vi "DB_MAIN.vi"(11 "Message Queues":T1) -> ()   [LabVIEW 2024]
uses:
  ARCH/Message Queue/All Message Queues.ctl
  ARCH/Message Queue/Message Cluster.ctl
  CAM/SRC/CTRLS/CAM module Data.ctl
  CTRLS/Main Tabs.ctl
  CTRLS/Serials DB Operations Enum.ctl
  CTRLS/Serial status Enum.ctl
  CTRLS/run statistics.ctl
  CTRLS/Workorder DB operation enum.ctl
  CTRLS/Workorder status enum.ctl
  CTRLS/Open Batch Data.ctl
  CTRLS/GLB_VAR.vi
  ARCH/Message Queue/Message Queue.lvlib
  Printer/Domino LM.lvlib
  CAM/RSeries_CAM.lvlib
panel:
  out "error out":errorcluster
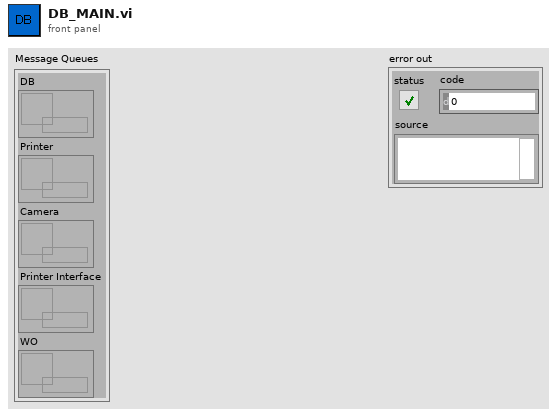
[diagram p1: front panel]
types:
  T1 = typedef "All Message Queues.ctl" = cluster{"DB":refnum<queue>, "Printer":refnum<queue>, "Camera":refnum<queue>, "Printer Interface":refnum<queue>, "WO":refnum<queue>}
  T2 = typedef "Message Queue.lvlib/Message Cluster.ctl" = cluster{"Message":string, "Message Data":variant}
  T3 = typedef "CAM module Data.ctl" = cluster{"IP":string, "sending Port ":u32, "BatchData":refnum<vi>, "Recieveing Port":u32, "Caller Quue":refnum<queue>}
  T4 = cluster{"Subscriber Message":string, "Subscribe Queue":refnum<queue>}
  T5 = typedef "Main Tabs.ctl" = enum32{"Login", "Main", "woManagement", "Settings", "Home"}
  T6 = enum8{"Enabled", "Disabled", "Disabled and Grayed Out"}
  T7 = enum16{"Init SRL Buffer", "Insert SRL in Buffer", "Insert SRL Status", "Remove SRL from Buffer", "pop serial"}
  T8 = typedef "Serial status Enum.ctl" = enum16{"NOT USED", "PRINTED", "ACCEPTED", "REJECTED"}
  T9 = typedef "Serials DB Operations Enum.ctl" = enum16{"Update serial verify status", "Get serials Based on Status", "Insert serials", "Update serial print status", "Get all Batch Serials", "Get Serial Status"}
  T10 = enum16{"Init SRL Buffer", "Insert SRL in Buffer", "Insert SRL Status", "Remove SRL from Buffer"}
  T11 = typedef "run statistics.ctl" = cluster{"Good":dbl, "Bad":dbl, "Good %":dbl, "Bad %":dbl}
  T12 = typedef "Workorder DB operation enum.ctl" = enum16{"Get Open Workorder", "Change WO Status", "Create WO", "Get ready and paused WOs"}
  T13 = typedef "Workorder status enum.ctl" = enum16{"Open", "Ready", "On Hold", "Closed"}
  T14 = typedef "Open Batch Data.ctl" = cluster{"Batch Name":string, "Batch Number":string, "GTIN":string, "Expiry Date":string, "MFG Date":string}
  T15 = typedef "REF.ctl" = cluster{"Save Settings":refnum<vi>, "Navigation":refnum<vi>, "Main Tab":refnum<vi>, "Password":refnum<vi>, "BatchData":refnum<vi>, "Serial Data":refnum<vi>, "Username":refnum<vi>, "Stop Printing":refnum<vi>, "Run statistics":refnum<vi>, "System settings":refnum<vi>, "Batch Managment contol":refnum<vi>, "Start Printing":refnum<vi>, "BatchData MNG":refnum<vi>, "MSG Cenetr":refnum<vi>, "Printer status":refnum<vi>, "Printer Message Config":refnum<vi>, "Ready and Paused Batches":refnum<vi>, "Camera Setup":refnum<vi>, "Batch statistics":refnum<vi>, "Logout":refnum<vi>}
  T16 = typedef "System settings.ctl" = cluster{"Machine IP":string, "Camera IP":string, "Printer IP":string, "Scanner settings":string, "Server Path":path, "Sending Port":u32, "Recieveing Port":u32}
  T17 = cluster{"DM Text":string, "GTIN":string, "Batch":string, "Expiry Date":string, "MFG Date":string, "Serial Number":string, "SSCC":string}
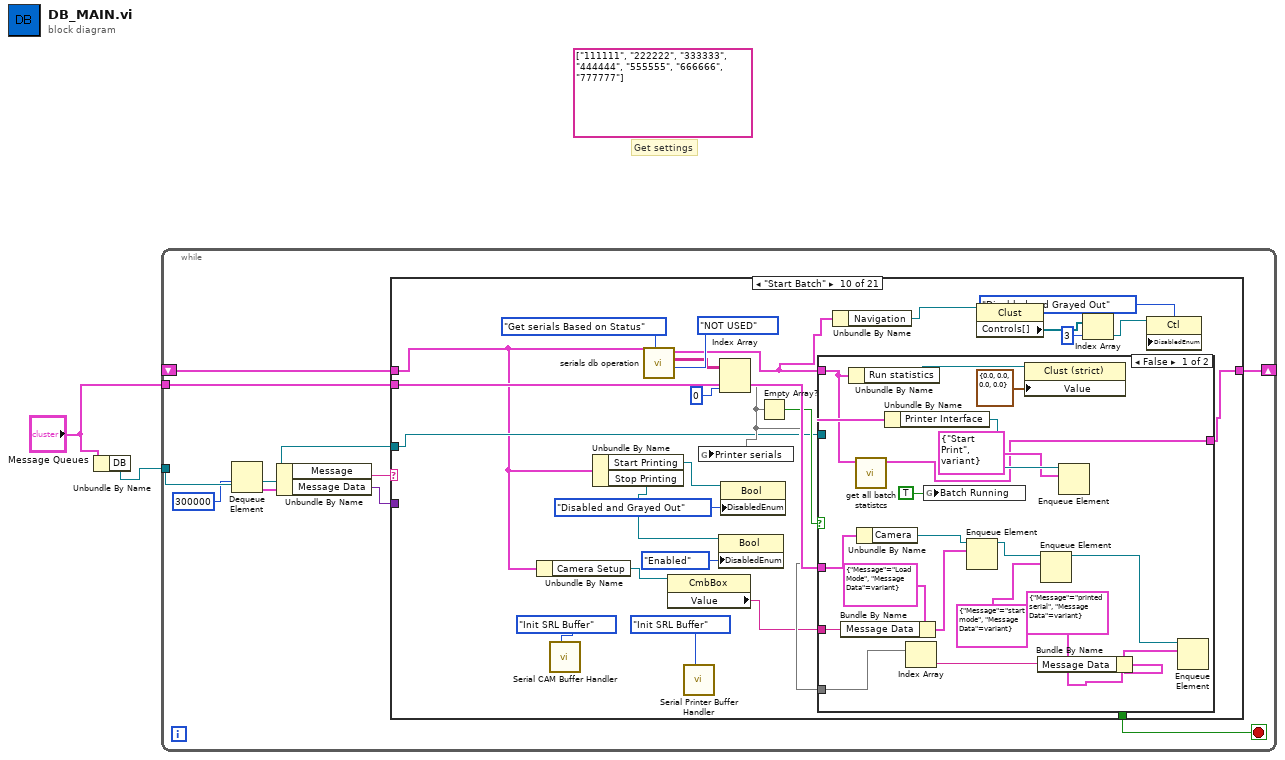
[diagram p0: block diagram]
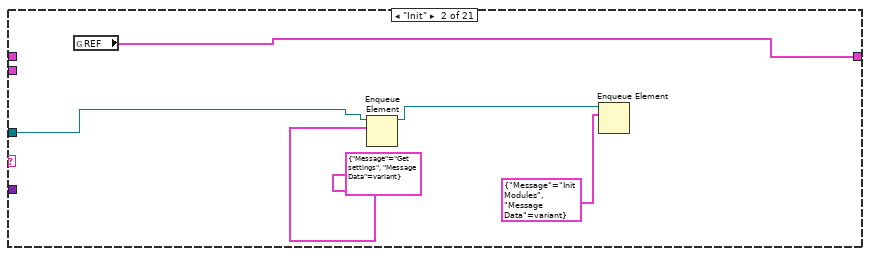
[diagram p3: hidden frame]
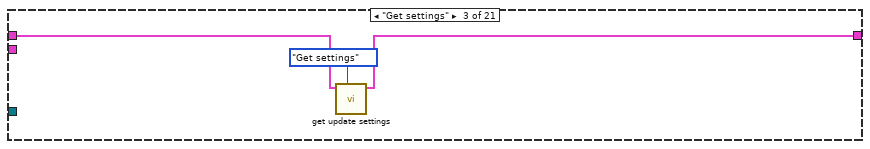
[diagram p4: hidden frame]
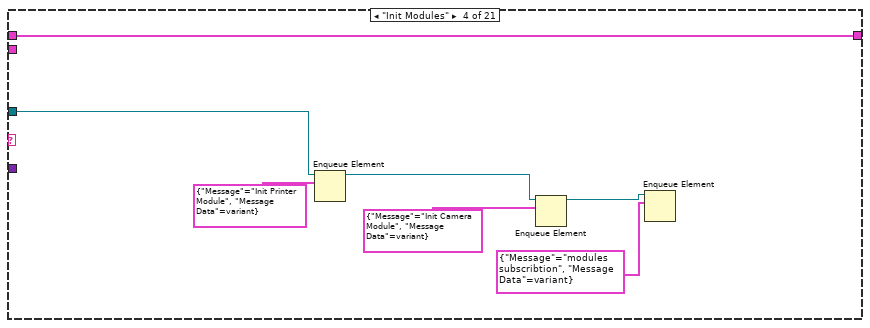
[diagram p5: hidden frame]
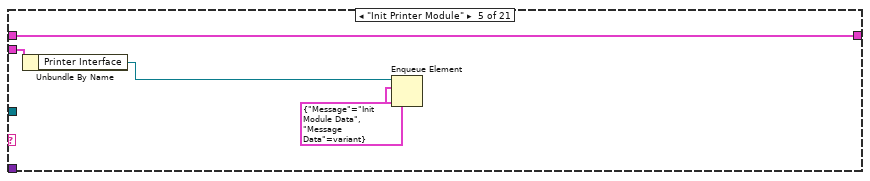
[diagram p6: hidden frame]
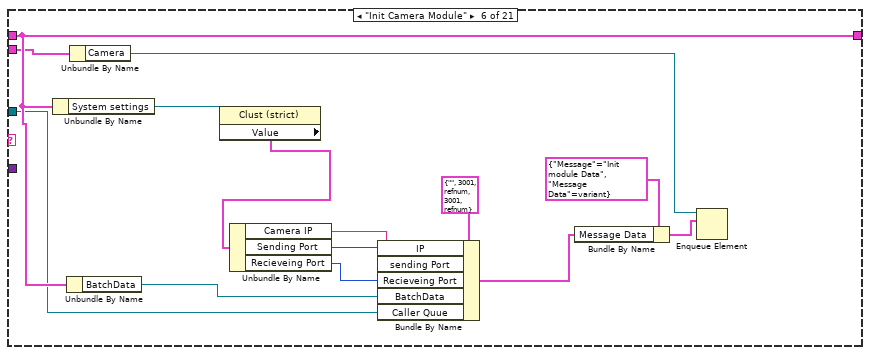
[diagram p7: hidden frame]
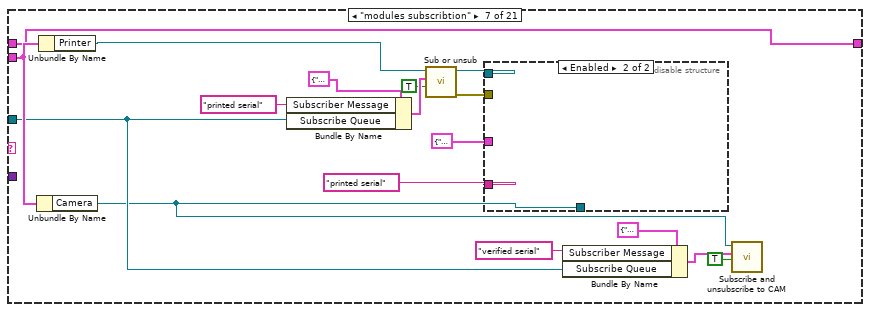
[diagram p8: hidden frame]
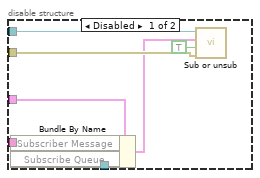
[diagram p9: hidden frame]
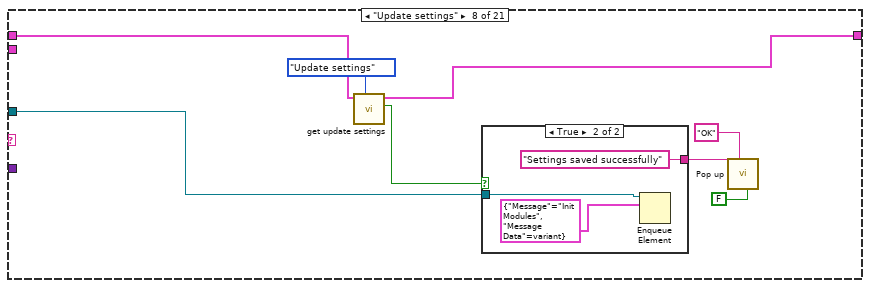
[diagram p10: hidden frame]
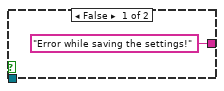
[diagram p11: hidden frame]
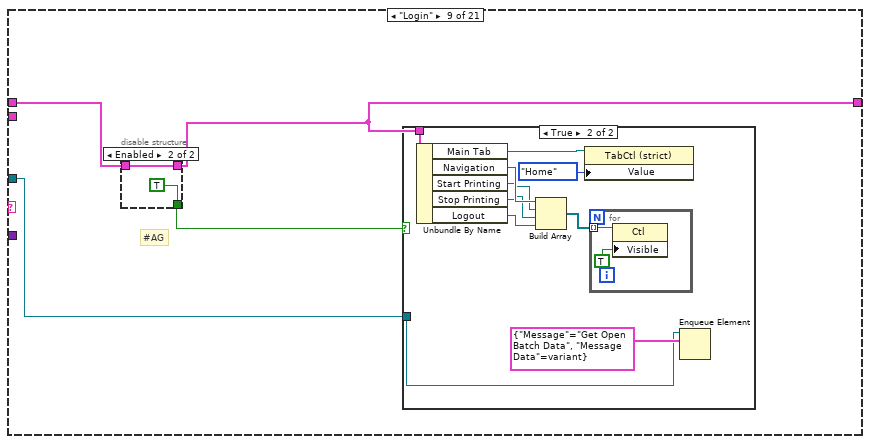
[diagram p12: hidden frame]
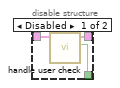
[diagram p13: hidden frame]
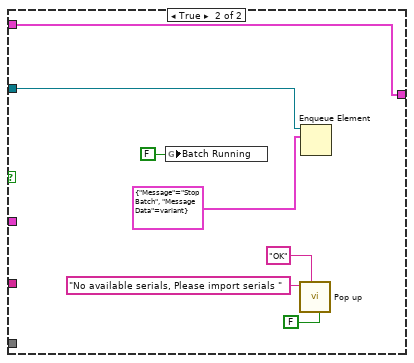
[diagram p15: hidden frame]
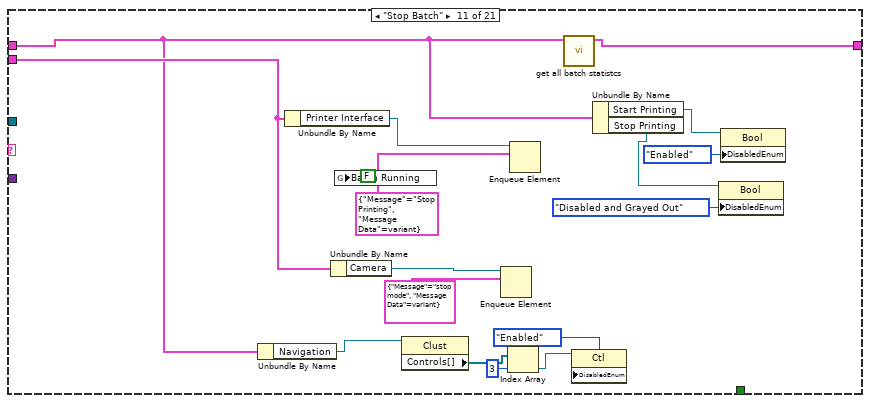
[diagram p16: hidden frame]
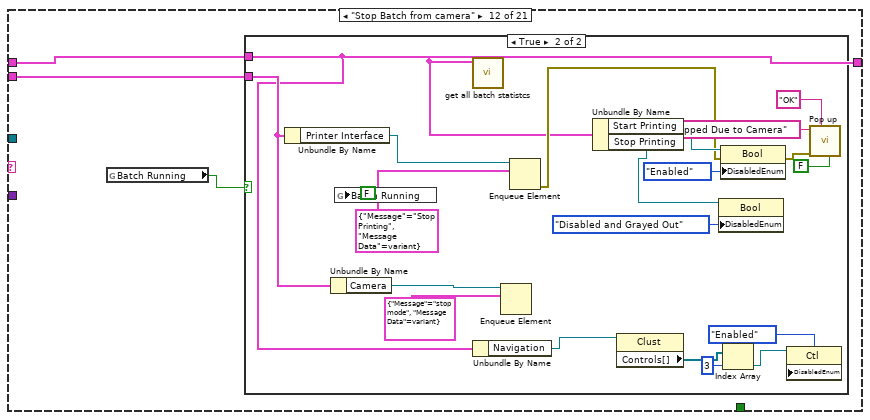
[diagram p17: hidden frame]
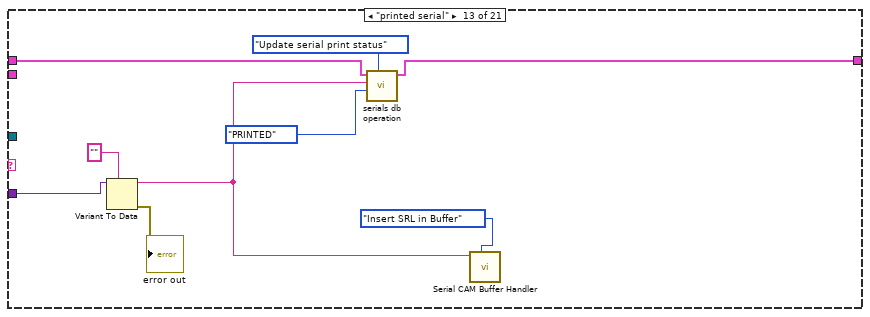
[diagram p19: hidden frame]
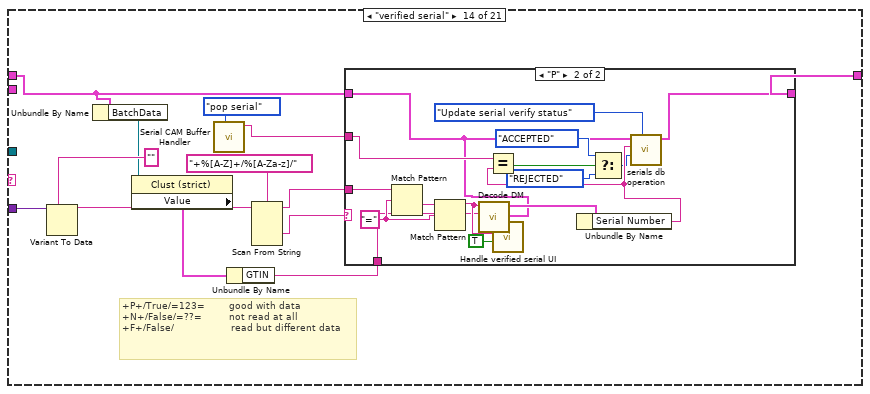
[diagram p20: hidden frame]
diagram:
  (unwired) string[] ["111111", "222222", "333333", "444444", "555555", "666666", "777777"] ("Printer serials")
  # "Get settings"
  n1 = Unbundle By Name("Message Queues") -> ("DB"=w2:refnum<queue>)
  n2 = while {
    tunnel: w2 -> [w12]
    tunnel: "Message Queues" -> [w5]
    shift-right: [w4] -> _
    shift-left: _ -> [w3]
    stop <- w7 stop-if-true
    n3 = Dequeue Element(queue=w12, timeout in ms (-1)=300000) -> (queue out=w8:refnum<queue>, element=w11:T2)  [unwired: 1 in, 2 out]
    n4 = Unbundle By Name(w11) -> ("Message"=w10:string, "Message Data"=w9:variant)
    n5 = case shown="\"Start Batch\"" w10 {
      tunnel: w9 -> [_ _ _ _ _ _ _ _ _ _ _ _ w199 w215 _ _ _ _ _ _ _]
      tunnel: w8 -> [_ w17 _ w28 _ w33 w49 w71 w86 w114 _ _ _ _ _ w275 _ w321 w340 w351 _]
      tunnel: [_ _ _ _ _ _ _ _ _ _ _ _ _ _ _ _ _ _ _ _ TRUE] -> w7
      tunnel: w5 -> [_ _ _ _ w32 w35 w54 _ _ w121 w155 w173 _ _ _ _ _ _ _ _ _]
      tunnel: [w13 w14 w20 w22 w29 w39 w53 w77 w84 w110 w161 w172 w202 w210 w264 w280 w306 w322 w344 w354 w360] -> w4
      tunnel: w3 -> [w13 _ w21 w22 w29 w39 w53 w78 w85 w113 w154 w172 w203 w207 w272 w278 w305 w320 w346 w353 w360]
      frame Default {
      }
      frame "Init" {
        n6 = global read "GLB_VAR.vi" "REF"() -> (w14:T15)
        n7 = Enqueue Element(queue=w17, element=T2 {"Message"="Get settings", "Message Data"=variant}) -> (queue out=w15:refnum<queue>)  [unwired: 2 in, 2 out]
        n8 = Enqueue Element(queue=w15, element=T2 {"Message"="Init Modules", "Message Data"=variant}) -> ()  [unwired: 2 in, 3 out]
      }
      frame "Get settings" {
        n9 = call "get update settings.vi"("settings DB OP"=enum16{"Get settings", "Update settings"}."Get settings", "REF in"=w21) -> ("REF out"=w20:T15)  [unwired: 7 in, 2 out]
      }
      frame "Init Modules" {
        n10 = Enqueue Element(queue=w28, element=T2 {"Message"="Init Printer Module", "Message Data"=variant}) -> (queue out=w25:refnum<queue>)  [unwired: 2 in, 2 out]
        n11 = Enqueue Element(queue=w25, element=T2 {"Message"="Init Camera Module", "Message Data"=variant}) -> (queue out=w24:refnum<queue>)  [unwired: 2 in, 2 out]
        n12 = Enqueue Element(queue=w24, element=T2 {"Message"="modules subscribtion", "Message Data"=variant}) -> ()  [unwired: 2 in, 3 out]
      }
      frame "Init Printer Module" {
        n13 = Unbundle By Name(w32) -> ("Printer Interface"=w31:refnum<queue>)
        n14 = Enqueue Element(queue=w31, element=T2 {"Message"="Init Module Data", "Message Data"=variant}) -> ()  [unwired: 2 in, 3 out]
      }
      frame "Init Camera Module" {
        n15 = Unbundle By Name(w39) -> ("System settings"=w41:refnum<vi>)
        n16 = Unbundle By Name(w39) -> ("BatchData"=w37:refnum<vi>)
        n17 = Unbundle By Name(w35) -> ("Camera"=w34:refnum<queue>)
        n18 = property class="Clust (strict)"(reference=w41) -> ("Value"=w40:T16)  [unwired: 1 in, 2 out]
        n19 = Unbundle By Name(w40) -> ("Camera IP"=w43:string, "Sending Port"=w44:u32, "Recieveing Port"=w36:u32)
        n20 = Bundle By Name(cluster=T3 {"IP"="", "sending Port "=3001, "BatchData"=refnum, "Recieveing Port"=3001, "Caller Quue"=refnum} ("CAM module Data"), "IP"=w43, "sending Port"=w44, "Recieveing Port"=w36, "BatchData"=w37, "Caller Quue"=w33) -> (w42:T3)
        n21 = Bundle By Name(cluster=T2 {"Message"="Init module Data", "Message Data"=variant} ("element"), "Message Data"=w42) -> (w45:T2)
        n22 = Enqueue Element(queue=w34, element=w45) -> ()  [unwired: 2 in, 3 out]
      }
      frame "modules subscribtion" {
        n23 = Unbundle By Name(w54) -> ("Camera"=w48:refnum<queue>)
        n24 = Unbundle By Name(w54) -> ("Printer"=w55:refnum<queue>)
        n25 = Bundle By Name(cluster=T4 {"Subscriber Message"="", "Subscribe Queue"=refnum} ("Subscriber Data"), "Subscriber Message"="printed serial", "Subscribe Queue"=w49) -> (w62:T4)
        n26 = call "Sub or unsub.vi"("Sub T/ Unsub F"=TRUE, "Subscriber Data"=w62, "Printer"=w55) -> ("error out"=w58:errorcluster, "printer queue out"=w57:refnum<queue>)  [unwired: 7 in]
        n27 = disable-structure shown="Enabled" {
          disable-tunnel: "printed serial" ("Subscriber Message") -> [w70 _]
          disable-tunnel: w58 -> [w69 _]
          disable-tunnel: w57 -> [w68 _]
          disable-tunnel: T4 {"Subscriber Message"="", "Subscribe Queue"=refnum} ("Subscriber Data") -> [w66 _]
          disable-tunnel: w48 -> [w65 _]
          frame Disabled {
            n28 = Bundle By Name(cluster=w66, "Subscriber Message"=w70, "Subscribe Queue"=w65) -> (w67:T4)
            n29 = call "Sub or unsub.vi"("error in (no error)"=w69, "Sub T/ Unsub F"=TRUE, "Subscriber Data"=w67, "Printer"=w68) -> ()  [unwired: 6 in, 2 out]
          }
          frame Enabled {
          }
        }
        n30 = Bundle By Name(cluster=T4 {"Subscriber Message"="", "Subscribe Queue"=refnum} ("Subscriber Data"), "Subscriber Message"="verified serial", "Subscribe Queue"=w49) -> (w50:T4)
        n31 = call "Subscribe and unsubscribe to CAM.vi"("Sub T/ Unsub F"=TRUE, "Subscriber Data"=w50, "Camera Queue"=w48) -> ()  [unwired: 7 in, 2 out]
      }
      frame "Update settings" {
        n32 = call "get update settings.vi"("settings DB OP"=enum16{"Get settings", "Update settings"}."Update settings", "REF in"=w78) -> ("success?"=w75:bool, "REF out"=w77:T15)  [unwired: 7 in, 1 out]
        n33 = case shown="True" w75 {
          tunnel: ["Error while saving the settings!" "Settings saved successfully"] -> w72
          tunnel: w71 -> [_ w80]
          frame False {
          }
          frame True {
            n34 = Enqueue Element(queue=w80, element=T2 {"Message"="Init Modules", "Message Data"=variant}) -> ()  [unwired: 2 in, 3 out]
          }
        }
        n35 = call "Pop up.vi"("Close Visible"=FALSE, "OK Boolean Text"="OK", "Title IN"=w72) -> ()  [unwired: 7 in, 2 out]
      }
      frame "Login" {
        # "#AG"
        n36 = disable-structure shown="Enabled" {
          disable-tunnel: w85 -> [w89 w91]
          disable-tunnel: [w88 w91] -> w84
          disable-tunnel: [w87 TRUE ("Result")] -> w83
          frame Disabled {
            n37 = call "handle user check.vi"("REF"=w89) -> ("Result"=w87:bool, "REF out"=w88:T15)  [unwired: 8 in, 1 out]
          }
          frame Enabled {
          }
        }
        n38 = case shown="True" w83 {
          tunnel: w84 -> [_ w100]
          tunnel: w86 -> [_ w97]
          frame False {
          }
          frame True {
            n39 = Unbundle By Name(w100) -> ("Main Tab"=w99:refnum<vi>, "Navigation"=w96:refnum<vi>, "Start Printing"=w95:refnum<vi>, "Stop Printing"=w94:refnum<vi>, "Logout"=w93:refnum<vi>)
            n40 = Build Array(w96, w95, w94, w93) -> (w92:refnum<vi>[])
            n41 = property on="Property Node" class="TabCtl (strict)"(reference=w99, "Value"=Main_Tabs."Home" ("Main Tab")) -> ()  [unwired: 1 in, 2 out]
            n42 = for {
              tunnel: w92 -> [w102] mode=indexing
              n43 = property on="Property Node" class="Ctl"(reference=w102, "Visible"=TRUE) -> ()  [unwired: 1 in, 2 out]
            }
            n44 = Enqueue Element(queue=w97, element=T2 {"Message"="Get Open Batch Data", "Message Data"=variant}) -> ()  [unwired: 2 in, 3 out]
          }
        }
      }
      frame "Start Batch" {
        n45 = Unbundle By Name(w113) -> ("Camera Setup"=w112:refnum<vi>)
        n46 = call "Serial CAM Buffer Handler.vi"("Serials buffer operations"=T7."Init SRL Buffer") -> ()  [unwired: 8 in, 3 out]
        n47 = Unbundle By Name(w113) -> ("Start Printing"=w120:refnum<vi>, "Stop Printing"=w118:refnum<vi>)
        n48 = call "serials db operation.vi"("SRL DB OP"=Serials_DB_Operations_Enum."Get serials Based on Status", "Status"=Serial_status_Enum."NOT USED", "REF"=w113) -> ("Fetched Serials"=w124:string[][], "REF out"=w109:T15)  [unwired: 5 in, 2 out]
        n49 = property class="CmbBox"(reference=w112) -> ("Value"=w111:string)  [unwired: 1 in, 2 out]
        n50 = call "Serial Printer Buffer Handler.vi"("Serials buffer operations"=T10."Init SRL Buffer") -> ()  [unwired: 9 in, 2 out]
        n51 = property class="Bool"(reference=w118, "DisabledEnum"=T6."Enabled" ("Disabled")) -> ()  [unwired: 1 in, 2 out]
        n52 = Index Array(array=w124, index (col)=0 ("disabled index (col)")) -> (element=w116:string[])  [unwired: 1 in]
        n53 = global write "GLB_VAR.vi" "Printer serials"(w116) -> ()
        n54 = property class="Bool"(reference=w120, "DisabledEnum"=T6."Disabled and Grayed Out" ("Disabled")) -> ()  [unwired: 1 in, 2 out]
        n55 = Empty Array?(array=w116) -> (empty?=w115:bool)
        n56 = case shown="False" w115 {
          tunnel: w116 -> [w141 _]
          tunnel: w121 -> [w138 _]
          tunnel: w109 -> [w129 w147]
          tunnel: w114 -> [_ w152]
          tunnel: w111 -> [w130 _]
          tunnel: [w128 w147] -> w110
          frame False {
            n57 = Bundle By Name(cluster=T2 {"Message"="Load Mode", "Message Data"=variant} ("element"), "Message Data"=w130) -> (w131:T2)
            n58 = Unbundle By Name(w129) -> ("Run statistics"=w135:refnum<vi>)
            n59 = call "get all batch statistcs.vi"("ref in"=w129) -> ("ref out"=w128:T15)  [unwired: 10 in]
            n60 = Unbundle By Name(w138) -> ("Camera"=w133:refnum<queue>)
            n61 = Unbundle By Name(w138) -> ("Printer Interface"=w146:refnum<queue>)
            n62 = Index Array(array=w141) -> (element=w140:string)  [unwired: 1 in]
            n63 = global write "GLB_VAR.vi" "Batch Running"(TRUE ("Batch Running")) -> ()
            n64 = Enqueue Element(queue=w133, element=w131) -> (queue out=w134:refnum<queue>)  [unwired: 2 in, 2 out]
            n65 = property class="Clust (strict)"(reference=w135, "Value"=T11 {"Good"=0.0, "Bad"=0.0, "Good %"=0.0, "Bad %"=0.0}) -> ()  [unwired: 1 in, 2 out]
            n66 = Bundle By Name(cluster=T2 {"Message"="printed serial", "Message Data"=variant} ("element"), "Message Data"=w140) -> (w139:T2)
            n67 = Enqueue Element(queue=w134, element=T2 {"Message"="start mode", "Message Data"=variant}) -> (queue out=w137:refnum<queue>)  [unwired: 2 in, 2 out]
            n68 = Enqueue Element(queue=w146, element=T2 {"Message"="Start Print", "Message Data"=variant}) -> ()  [unwired: 2 in, 3 out]
            n69 = Enqueue Element(queue=w137, element=w139) -> ()  [unwired: 2 in, 3 out]
          }
          frame True {
            n70 = global write "GLB_VAR.vi" "Batch Running"(FALSE ("Batch Running")) -> ()
            n71 = call "Pop up.vi"("Close Visible"=FALSE, "OK Boolean Text"="OK", "Title IN"="No available serials, Please import serials ") -> ()  [unwired: 7 in, 2 out]
            n72 = Enqueue Element(queue=w152, element=T2 {"Message"="Stop Batch", "Message Data"=variant}) -> ()  [unwired: 2 in, 3 out]
          }
        }
        n73 = Unbundle By Name(w109) -> ("Navigation"=w108:refnum<vi>)
        n74 = property class="Clust"(reference=w108) -> ("Controls[]"=w107:refnum<vi>[])  [unwired: 1 in, 2 out]
        n75 = Index Array(array=w107, index=3) -> (element=w105:refnum<vi>)
        n76 = property class="Ctl"(reference=w105, "DisabledEnum"=T6."Disabled and Grayed Out" ("Disabled")) -> ()  [unwired: 1 in, 2 out]
      }
      frame "Stop Batch" {
        n77 = Unbundle By Name(w154) -> ("Navigation"=w160:refnum<vi>)
        n78 = Unbundle By Name(w155) -> ("Printer Interface"=w170:refnum<queue>)
        n79 = Unbundle By Name(w155) -> ("Camera"=w167:refnum<queue>)
        n80 = global write "GLB_VAR.vi" "Batch Running"(FALSE ("Batch Running")) -> ()
        n81 = property class="Clust"(reference=w160) -> ("Controls[]"=w159:refnum<vi>[])  [unwired: 1 in, 2 out]
        n82 = Enqueue Element(queue=w167, element=T2 {"Message"="stop mode", "Message Data"=variant}) -> ()  [unwired: 2 in, 3 out]
        n83 = Index Array(array=w159, index=3) -> (element=w157:refnum<vi>)
        n84 = Enqueue Element(queue=w170, element=T2 {"Message"="Stop Printing", "Message Data"=variant}) -> ()  [unwired: 2 in, 3 out]
        n85 = call "get all batch statistcs.vi"("ref in"=w154) -> ("ref out"=w161:T15)  [unwired: 10 in]
        n86 = property class="Ctl"(reference=w157, "DisabledEnum"=T6."Enabled" ("Disabled")) -> ()  [unwired: 1 in, 2 out]
        n87 = Unbundle By Name(w154) -> ("Start Printing"=w162:refnum<vi>, "Stop Printing"=w164:refnum<vi>)
        n88 = property class="Bool"(reference=w164, "DisabledEnum"=T6."Disabled and Grayed Out" ("Disabled")) -> ()  [unwired: 1 in, 2 out]
        n89 = property class="Bool"(reference=w162, "DisabledEnum"=T6."Enabled" ("Disabled")) -> ()  [unwired: 1 in, 2 out]
      }
      frame "Stop Batch from camera" {
        n90 = global read "GLB_VAR.vi" "Batch Running"() -> (w171:bool)
        n91 = case shown="True" w171 {
          tunnel: w173 -> [_ w189]
          tunnel: w172 -> [_ w174]
          frame False {
          }
          frame True {
            n92 = Unbundle By Name(w189) -> ("Printer Interface"=w194:refnum<queue>)
            n93 = Unbundle By Name(w189) -> ("Camera"=w191:refnum<queue>)
            n94 = global write "GLB_VAR.vi" "Batch Running"(FALSE ("Batch Running")) -> ()
            n95 = call "get all batch statistcs.vi"("ref in"=w174) -> ()  [unwired: 10 in, 1 out]
            n96 = Unbundle By Name(w174) -> ("Navigation"=w179:refnum<vi>)
            n97 = Enqueue Element(queue=w191, element=T2 {"Message"="stop mode", "Message Data"=variant}) -> ()  [unwired: 2 in, 3 out]
            n98 = Enqueue Element(queue=w194, element=T2 {"Message"="Stop Printing", "Message Data"=variant}) -> (error out=w184:errorcluster)  [unwired: 2 in, 2 out]
            n99 = Unbundle By Name(w174) -> ("Start Printing"=w185:refnum<vi>, "Stop Printing"=w187:refnum<vi>)
            n100 = property class="Clust"(reference=w179) -> ("Controls[]"=w178:refnum<vi>[])  [unwired: 1 in, 2 out]
            n101 = property class="Bool"(reference=w187, "DisabledEnum"=T6."Disabled and Grayed Out" ("Disabled")) -> ()  [unwired: 1 in, 2 out]
            n102 = property class="Bool"(reference=w185, error in=w184, "DisabledEnum"=T6."Enabled" ("Disabled")) -> (error out=w183:errorcluster)  [unwired: 1 out]
            n103 = Index Array(array=w178, index=3) -> (element=w176:refnum<vi>)
            n104 = property class="Ctl"(reference=w176, "DisabledEnum"=T6."Enabled" ("Disabled")) -> ()  [unwired: 1 in, 2 out]
            n105 = call "Pop up.vi"("Close Visible"=FALSE, "OK Boolean Text"="OK", "error in (no error)"=w183, "Title IN"="Printing Stopped Due to Camera") -> ()  [unwired: 6 in, 2 out]
          }
        }
      }
      frame "printed serial" {
        n106 = Variant To Data(type="", Variant=w199) -> (data=w196:string, error out=→"error out":errorcluster)  [unwired: 1 in]
        n107 = call "serials db operation.vi"("SRL DB OP"=Serials_DB_Operations_Enum."Update serial print status", "Status"=Serial_status_Enum."PRINTED", "Serial"=w196, "REF"=w203) -> ("REF out"=w202:T15)  [unwired: 4 in, 3 out]
        n108 = call "Serial CAM Buffer Handler.vi"("Serials buffer operations"=T7."Insert SRL in Buffer", "Serial"=w196) -> ()  [unwired: 7 in, 3 out]
      }
      frame "verified serial" {
        # "+P+/True/=123=        good with data\n+N+/False/=??=         not read at all\n+F+/False/                   read but different data"
        n109 = Variant To Data(type="", Variant=w215) -> (data=w212:string)  [unwired: 1 in, 1 out]
        n110 = Unbundle By Name(w207) -> ("BatchData"=w206:refnum<vi>)
        n111 = property class="Clust (strict)"(reference=w206) -> ("Value"=w205:T14)  [unwired: 1 in, 2 out]
        n112 = call "Serial CAM Buffer Handler.vi"("Serials buffer operations"=T7."pop serial") -> ("poped serial"=w208:string)  [unwired: 8 in, 2 out]
        n113 = Unbundle By Name(w205) -> ("GTIN"=w204:string)
        n114 = Scan From String(format string="+%[A-Z]+/%[A-Za-z]/", input string=w212) -> (remaining string=w213:string, output 1=w214:string)  [unwired: 5 in, 2 out]
        n115 = case shown="\"P\"" w214 {
          tunnel: w213 -> [w217 w239]
          tunnel: [w222 w236] -> w210
          tunnel: w207 -> [w219 w225]
          tunnel: w208 -> [w221 w233]
          tunnel: w204 -> [_ w224]
          frame Default {
            n116 = call "Handle verified serial UI.vi"("serial status"=FALSE, "DataMatrix Text"=w217, "REF in"=w219) -> ()  [unwired: 8 in, 1 out]
            n117 = call "serials db operation.vi"("SRL DB OP"=Serials_DB_Operations_Enum."Update serial verify status", "Status"=Serial_status_Enum."REJECTED", "Serial"=w221, "REF"=w219) -> ("REF out"=w222:T15)  [unwired: 4 in, 3 out]
          }
          frame "P" {
            w237 = "=" ("regular expression")
            n118 = Match Pattern(string=w239, regular expression=w237) -> (after substring=w238:string)  [unwired: 1 in, 3 out]
            n119 = Match Pattern(string=w238, regular expression=w237) -> (before substring=w227:string)  [unwired: 1 in, 3 out]
            n120 = call "Decode DM.vi"("GTIN"=w224, "DataMatrix Text"=w227) -> ("DM CONTENT OUT"=w234:T17)  [unwired: 9 in]
            n121 = call "Handle verified serial UI.vi"("serial status"=TRUE, "DataMatrix Text"=w227, "REF in"=w225) -> ()  [unwired: 8 in, 1 out]
            n122 = Unbundle By Name(w234) -> ("Serial Number"=w232:string)
            n123 = Equal?(x=w233, y=w232) -> (x = y?=w231:bool)
            n124 = Select(t=Serial_status_Enum."ACCEPTED" ("Status"), s=w231, f=Serial_status_Enum."REJECTED" ("Status")) -> (s? t:f=w228:T8)
            n125 = call "serials db operation.vi"("SRL DB OP"=Serials_DB_Operations_Enum."Update serial verify status", "Status"=w228, "Serial"=w232, "REF"=w225) -> ("REF out"=w236:T15)  [unwired: 4 in, 3 out]
          }
        }
      }
      frame "Get Open Batch Data" {
        n126 = call "Workorder DB Operation.vi"("WO OP"=Workorder_DB_operation_enum."Get Open Workorder", "REF in"=w272) -> ("Open batch"=w268:T14, "REF out"=w266:T15)  [unwired: 5 in, 3 out]
        n127 = Unbundle By Name(w266) -> ("BatchData MNG"=w269:refnum<vi>, "Batch Managment contol"=w256:refnum<vi>)
        n128 = Unbundle By Name(w268) -> ("Batch Name"=w267:string)
        n129 = Unbundle By Name(w266) -> ("BatchData"=w270:refnum<vi>)
        n130 = Empty String/Path?(string/path=w267) -> (empty?=w247:bool)
        n131 = property class="Clust (strict)"(reference=w270, "Value"=w268) -> ()  [unwired: 1 in, 2 out]
        n132 = Select(t=T6."Enabled" ("Disabled"), s=w247, f=T6."Disabled and Grayed Out" ("Disabled")) -> (s? t:f=w254:T6)
        n133 = Select(t=T6."Disabled and Grayed Out" ("Disabled"), s=w247, f=T6."Enabled" ("Disabled")) -> (s? t:f=w240:T6)
        n134 = property class="Clust (strict)"(reference=w269, "Value"=w268, "DisabledEnum"=w254) -> ()  [unwired: 1 in, 2 out]
        n135 = property class="Clust"(reference=w256) -> ("Controls[]"=w255:refnum<vi>[])  [unwired: 1 in, 2 out]
        n136 = call "Workorder DB Operation.vi"("WO OP"=Workorder_DB_operation_enum."Get ready and paused WOs", "REF in"=w266) -> ("REF out"=w264:T15, "paused and ready WOs"=w262:string[])  [unwired: 5 in, 3 out]
        n137 = Index Array(array=w255, index #1=2 ("index"), index #2=5 ("index"), index #3=0 ("index"), index #4=1 ("index"), index #5=3 ("index"), index #6=4 ("index")) -> (element #1=w252:refnum<vi>, element #2=w259:refnum<vi>, element #3=w244:refnum<vi>, element #4=w243:refnum<vi>, element #5=w242:refnum<vi>, element #6=w241:refnum<vi>)
        n138 = for {
          tunnel: w262 -> [w274] mode=indexing
          tunnel: [w273] -> w261 mode=indexing
          n139 = Bundle(w274, w274) -> (w273:cluster{string, string})  [unwired: 1 in]
        }
        n140 = Unbundle By Name(w264) -> ("Ready and Paused Batches"=w263:refnum<vi>)
        n141 = property class="Ctl"(reference=w259, "DisabledEnum"=w254) -> ()  [unwired: 1 in, 2 out]
        n142 = property class="Ctl"(reference=w244, "DisabledEnum"=w240) -> ()  [unwired: 1 in, 2 out]
        n143 = property class="Ctl"(reference=w252, "DisabledEnum"=w254) -> ()  [unwired: 1 in, 2 out]
        n144 = property class="CmbBox"(reference=w263, "Strings And Values[]"=w261) -> ()  [unwired: 1 in, 2 out]
        n145 = property class="Ctl"(reference=w243, "DisabledEnum"=w240) -> ()  [unwired: 1 in, 2 out]
        n146 = property class="Ctl"(reference=w241, "DisabledEnum"=w240) -> ()  [unwired: 1 in, 2 out]
        n147 = property class="Ctl"(reference=w242, "DisabledEnum"=w240) -> ()  [unwired: 1 in, 2 out]
      }
      frame "Close Workorder" {
        n148 = call "Export serials.vi"("REF"=w278) -> ("Success?"=w276:bool, "REF OUT"=w277:T15)  [unwired: 8 in, 1 out]
        n149 = case shown="False" w276 {
          tunnel: [w282 w285] -> w280
          tunnel: [errorcluster {"status"=TRUE, "code"=0, "source"=""} ("error out") w284] -> w279
          tunnel: w277 -> [w282 w283]
          frame False {
          }
          frame True {
            n150 = Unbundle By Name(w283) -> ("BatchData"=w289:refnum<vi>)
            n151 = property class="Clust (strict)"(reference=w289) -> ("Value"=w288:T14)  [unwired: 1 in, 2 out]
            n152 = Unbundle By Name(w288) -> ("Batch Name"=w287:string)
            n153 = call "Workorder DB Operation.vi"("WO OP"=Workorder_DB_operation_enum."Change WO Status", "Status"=Workorder_status_enum."Closed", "Workorder name"=w287, "REF in"=w283) -> ("error out"=w284:errorcluster, "REF out"=w285:T15)  [unwired: 3 in, 3 out]
          }
        }
        n154 = case shown="No Error" w279 {
          tunnel: w280 -> [w298 _]
          tunnel: w275 -> [w294 _]
          frame No Error {
            n155 = Enqueue Element(queue=w294, element=T2 {"Message"="Get Open Batch Data", "Message Data"=variant}) -> ()  [unwired: 2 in, 3 out]
            n156 = Unbundle By Name(w298) -> ("BatchData MNG"=w299:refnum<vi>)
            n157 = property class="Clust (strict)"(reference=w299, "Value"=T14 {"Batch Name"="", "Batch Number"="", "GTIN"="", "Expiry Date"="", "MFG Date"=""}, "DisabledEnum"=T6."Enabled" ("Disabled")) -> ()  [unwired: 1 in, 2 out]
            n158 = call "Pop up.vi"("Close Visible"=FALSE, "OK Boolean Text"="OK", "Title IN"="Batch closed Successfully") -> ()  [unwired: 7 in, 2 out]
          }
          frame Error {
            n159 = call "Pop up.vi"("Close Visible"=FALSE, "OK Boolean Text"="OK", "Title IN"="Faild to close batch") -> ()  [unwired: 7 in, 2 out]
          }
        }
      }
      frame "Export Rejected Serials" {
        n160 = call "Export Rejected serials.vi"("REF"=w305) -> ("Success?"=w303:bool, "REF OUT"=w304:T15)  [unwired: 8 in, 1 out]
        n161 = case shown="True" w303 {
          tunnel: [w310 w314] -> w306
          tunnel: w304 -> [w310 w314]
          frame False {
            n162 = call "Pop up.vi"("Close Visible"=FALSE, "OK Boolean Text"="OK", "Title IN"="Faild to export rejected serials") -> ()  [unwired: 7 in, 2 out]
          }
          frame True {
            n163 = call "Pop up.vi"("Close Visible"=FALSE, "OK Boolean Text"="OK", "Title IN"="Rejected Serials Exported Successfully") -> ()  [unwired: 7 in, 2 out]
          }
        }
      }
      frame "Open Workorder" {
        n164 = call "Workorder DB Operation.vi"("WO OP"=Workorder_DB_operation_enum."Get Open Workorder", "REF in"=w320) -> ("Open batch"=w316:T14, "REF out"=w319:T15)  [unwired: 5 in, 3 out]
        n165 = Unbundle By Name(w316) -> ("Batch Name"=w317:string)
        n166 = Empty String/Path?(string/path=w317) -> (empty?=w315:bool)
        n167 = case shown="False" w315 {
          tunnel: w319 -> [w326 w334]
          tunnel: [w326 w331] -> w322
          tunnel: w321 -> [_ w329]
          frame False {
            n168 = call "Pop up.vi"("Close Visible"=FALSE, "OK Boolean Text"="OK", "Title IN"="You already have an open batch, Close the open batch first") -> ()  [unwired: 7 in, 2 out]
          }
          frame True {
            n169 = Unbundle By Name(w334) -> ("Ready and Paused Batches"=w333:refnum<vi>)
            n170 = Enqueue Element(queue=w329, element=T2 {"Message"="Get Open Batch Data", "Message Data"=variant}) -> ()  [unwired: 2 in, 3 out]
            n171 = property class="CmbBox"(reference=w333) -> ("Value"=w327:string)  [unwired: 1 in, 2 out]
            n172 = call "Workorder DB Operation.vi"("WO OP"=Workorder_DB_operation_enum."Change WO Status", "Status"=Workorder_status_enum."Open", "Workorder name"=w327, "REF in"=w334) -> ("error out"=w330:errorcluster, "REF out"=w331:T15)  [unwired: 3 in, 3 out]
            n173 = case shown="No Error" w330 {
              tunnel: w331 -> [w338 _]
              frame No Error {
                n174 = Unbundle By Name(w338) -> ("BatchData MNG"=w339:refnum<vi>)
                n175 = property class="Clust (strict)"(reference=w339, "Value"=T14 {"Batch Name"="", "Batch Number"="", "GTIN"="", "Expiry Date"="", "MFG Date"=""}, "DisabledEnum"=T6."Enabled" ("Disabled")) -> ()  [unwired: 1 in, 2 out]
              }
              frame Error {
              }
            }
          }
        }
      }
      frame "Create new WO" {
        n176 = Unbundle By Name(w346) -> ("BatchData MNG"=w345:refnum<vi>)
        n177 = property class="Clust (strict)"(reference=w345) -> ("Value"=w342:T14)  [unwired: 1 in, 2 out]
        n178 = Enqueue Element(queue=w340, element=T2 {"Message"="Get Open Batch Data", "Message Data"=variant}) -> ()  [unwired: 2 in, 3 out]
        n179 = call "Workorder DB Operation.vi"("create batch"=w342, "WO OP"=Workorder_DB_operation_enum."Create WO", "REF in"=w346) -> ("error out"=w343:errorcluster, "REF out"=w344:T15)  [unwired: 4 in, 3 out]
        n180 = case shown="No Error" w343 {
          tunnel: w344 -> [w349 _]
          frame No Error {
            n181 = Unbundle By Name(w349) -> ("BatchData MNG"=w350:refnum<vi>)
            n182 = property class="Clust (strict)"(reference=w350, "DisabledEnum"=T6."Disabled" ("Disabled")) -> ()  [unwired: 1 in, 2 out]
          }
          frame Error {
          }
        }
      }
      frame "Pause Workorder" {
        n183 = Unbundle By Name(w353) -> ("BatchData"=w358:refnum<vi>)
        n184 = Enqueue Element(queue=w351, element=T2 {"Message"="Get Open Batch Data", "Message Data"=variant}) -> ()  [unwired: 2 in, 3 out]
        n185 = property class="Clust (strict)"(reference=w358) -> ("Value"=w357:T14)  [unwired: 1 in, 2 out]
        n186 = Unbundle By Name(w357) -> ("Batch Name"=w356:string)
        n187 = call "Workorder DB Operation.vi"("WO OP"=Workorder_DB_operation_enum."Change WO Status", "Status"=Workorder_status_enum."On Hold", "Workorder name"=w356, "REF in"=w353) -> ("REF out"=w354:T15)  [unwired: 3 in, 4 out]
      }
      frame "Exit" {
      }
    }
  }
